vi "Practica3.3_Case.vi"() -> ()   [LabVIEW 2022 SP3]
panel:
  out "Valor aleatorio":dbl(knob) scale=0.0..10.0
  out "Es igual\nNo es igual":bool
  in  "Selección de valor":dbl
  # "Anahí Montserrat Vázquez Padilla \nPráctica 03: Case \n31/01/2024"
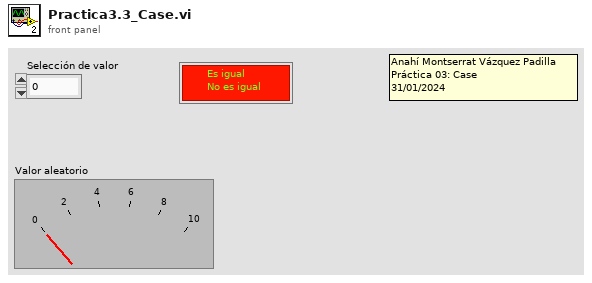
[diagram p1: front panel]
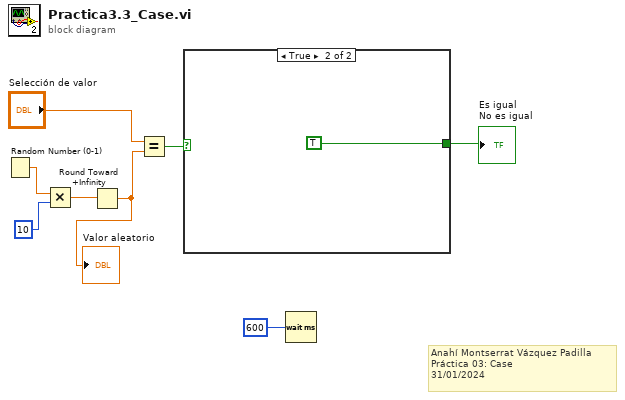
[diagram p0: block diagram]
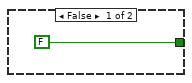
[diagram p2: hidden frame]
diagram:
  # "Anahí Montserrat Vázquez Padilla \nPráctica 03: Case \n31/01/2024"
  n1 = Random Number (0-1)() -> (number: 0 to 1=w8:dbl)
  n2 = Multiply(x=w8, y=10) -> (x*y=w6:dbl)
  n3 = Round Toward +Infinity(x=w6) -> (ceil(x): smallest int >= x=w1:dbl)
  "Valor aleatorio" <- w1
  n4 = Equal?(x="Selección de valor", y=w1) -> (x = y?=w4:bool)
  n5 = case shown="True" w4 {
    tunnel: [FALSE TRUE] -> w3
    frame False {
    }
    frame True {
    }
  }
  "Es igual\nNo es igual" <- w3
  n6 = Wait (ms)(milliseconds to wait=600) -> ()  [unwired: 1 out]
